vi "process.vi"(8 "error in (no error)":errorcluster, 11 "Server in":refnum<class "Server.lvclass">) -> (0 "error out":errorcluster)   [LabVIEW 2013, in "MQTT Server.lvlib" / "Server.lvclass"]
uses:
  Server.lvclass
  <vilib>/LabVIEW Open Source Project/MQTT Connection/MQTT_Base/Base Class/MQTT_Base.lvclass
  <vilib>/LabVIEW Open Source Project/MQTT Connection/MQTT_Base/Base Class/MQTT_Base.lvclass/MQTT_Base.ctl
  Server.lvclass/Server.ctl
  ConnectionHandler/ConnectionHandler.lvclass/ConnectionHandler.ctl
  ConnectionHandler/ConnectionHandler.lvclass
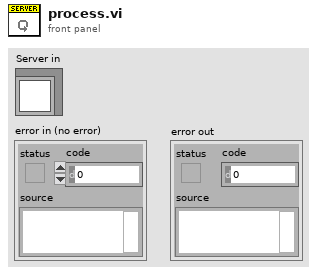
[diagram p1: front panel]
types:
  T1 = typedef "MQTT Base.lvlib/MQTT_Base.lvclass/Public Events -- cluster.ctl" = cluster{"Stop Event":refnum<user-event>, "Error Event":refnum<user-event>, "Inbound Message":refnum<user-event>}
  T2 = typedef "MQTT Server.lvlib/ConnectionHandler.lvclass/Public Events -- Cluster.ctl" = cluster{"NbConnections":refnum<user-event>}
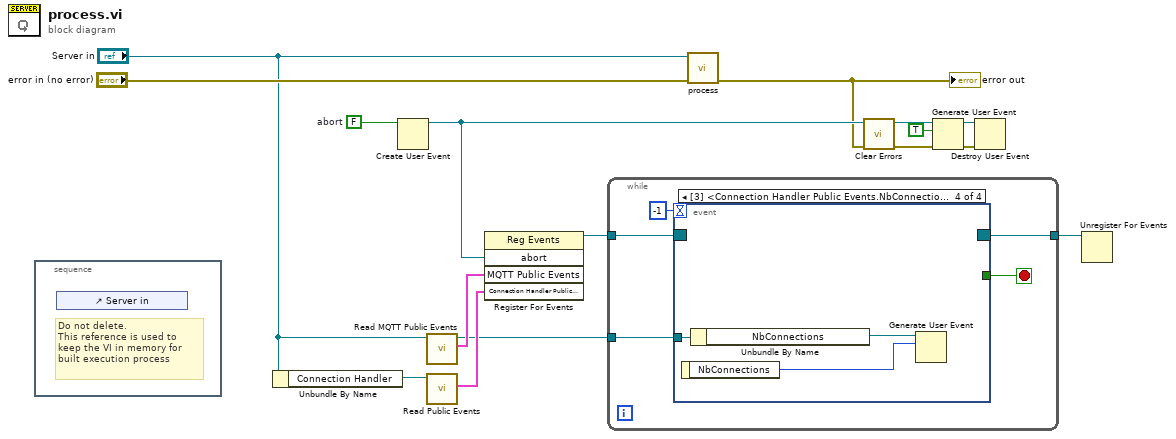
[diagram p0: block diagram]
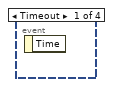
[diagram p2: hidden frame]
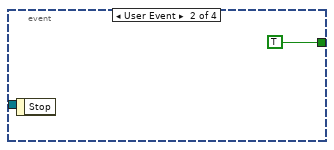
[diagram p3: hidden frame]
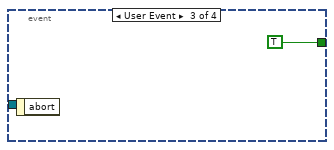
[diagram p4: hidden frame]
diagram:
  w11 = FALSE  # abort
  n1 = stacked-sequence {
    frame #0 {
      # "Do not delete.\nThis reference is used to keep the VI in memory for built execution process"
      n2 = control-ref of="Server in"() -> ()  [unwired: 1 out]
    }
  }
  n3 = Unbundle By Name("Server in") -> ("Connection Handler"=w12:refnum<class "ConnectionHandler.lvclass">)
  n4 = Create User Event(user event datatype=w11) -> (user event=w9:refnum<user-event>)  [unwired: 1 in, 1 out]
  n5 = call <vilib>:"Read MQTT Public Events.vi"("MQTT_Base in"="Server in") -> ("MQTT Public Events"=w14:T1, "MQTT_Base out"=w2:refnum<class "Server.lvclass">)  [unwired: 8 in, 1 out]
  n6 = call "Read Public Events.vi"("TCPConnectionHandler in"=w12) -> ("Connection Handler Public Events"=w3:T2)  [unwired: 8 in, 2 out]
  n7 = register-events(w9, w14, w3) -> (reference out=w10:refnum<event-registration>)  [unwired: 2 in, 1 out]
  n8 = while {
    tunnel: w10 -> [w19]
    tunnel: [w17] -> w4
    tunnel: w2 -> [w16]
    stop <- w18 stop-if-true
    n9 = event shown="[3] <Connection Handler Public Events.NbConnections>: User Event" {
      selector: w19 -> [_ _ _ _]
      dyn-events: [_ _ _ _] -> w17
      timeout: -1 -> [_ _ _ _]
      tunnel: [_ TRUE TRUE _] -> w18
      tunnel: w16 -> [_ _ _ w25]
      event Timeout {
        n10 = event-data() -> ()  [unwired: 1 in, 1 out]
      }
      event User Event {
        n11 = event-data() -> ()  [unwired: 1 in, 1 out]
      }
      event User Event {
        n12 = event-data() -> ()  [unwired: 1 in, 1 out]
      }
      event User Event {
        n13 = event-data() -> ("NbConnections"=w23:u32)  [unwired: 1 in]
        n14 = Unbundle By Name(w25) -> ("NbConnections"=w24:refnum<user-event>)
        n15 = Generate User Event(user event=w24, event data cluster=w23) -> ()  [unwired: 2 in, 2 out]
      }
    }
  }
  n16 = call-parent "process.vi"("error in (no error)"="error in (no error)", "MQTT_Base in"="Server in") -> ("error out"=w5:errorcluster)  [unwired: 9 in]
  "error out" <- w5
  n17 = call <vilib>:"Clear Errors.vi"("error in (no error)"=w5) -> ("error out"=w6:errorcluster)  [unwired: 6 in]
  n18 = Generate User Event(user event=w9, event data cluster=TRUE ("event data"), error in=w6) -> (user event out=w8:refnum<user-event>, error out=w7:errorcluster)  [unwired: 1 in]
  n19 = Destroy User Event(user event=w8, error in=w7) -> ()  [unwired: 1 out]
  n20 = Unregister For Events(event registration refnum=w4) -> ()  [unwired: 1 in, 1 out]
